vi "V3_IRCal.vi"() -> ()   [LabVIEW 2019]
uses:
  WSCbot_V3_Toolkit.lvlibp/WSCBOTV3_Toolkit/Sensor/LowLevel/IR_Chanel.ctl
  <vilib>/Platform/TimedLoop/XDataNode/timing_clust.ctl
  <vilib>/Platform/TimedLoop/XDataNode/nitl_modes.ctl
  <vilib>/Platform/TimedLoop/XDataNode/wakeup.ctl
  <vilib>/platform/TimedLoop/XDataNode/XDataNode.xnode
  WSCbot_V3_Toolkit.lvlibp
  <vilib>/Platform/TimedLoop/XDataNode/XDNodeRunTimeDep.lvlib
panel:
  out "x/y":dbl
  out "Waveform Chart 2":T1(graph)
  out "result":bool
  in  "P3":dbl
  in  "P2":dbl
  in  "P1":dbl
  out "Waveform Chart":T1(graph)
  in  "IR_Chanel":T2[](array[typedef])
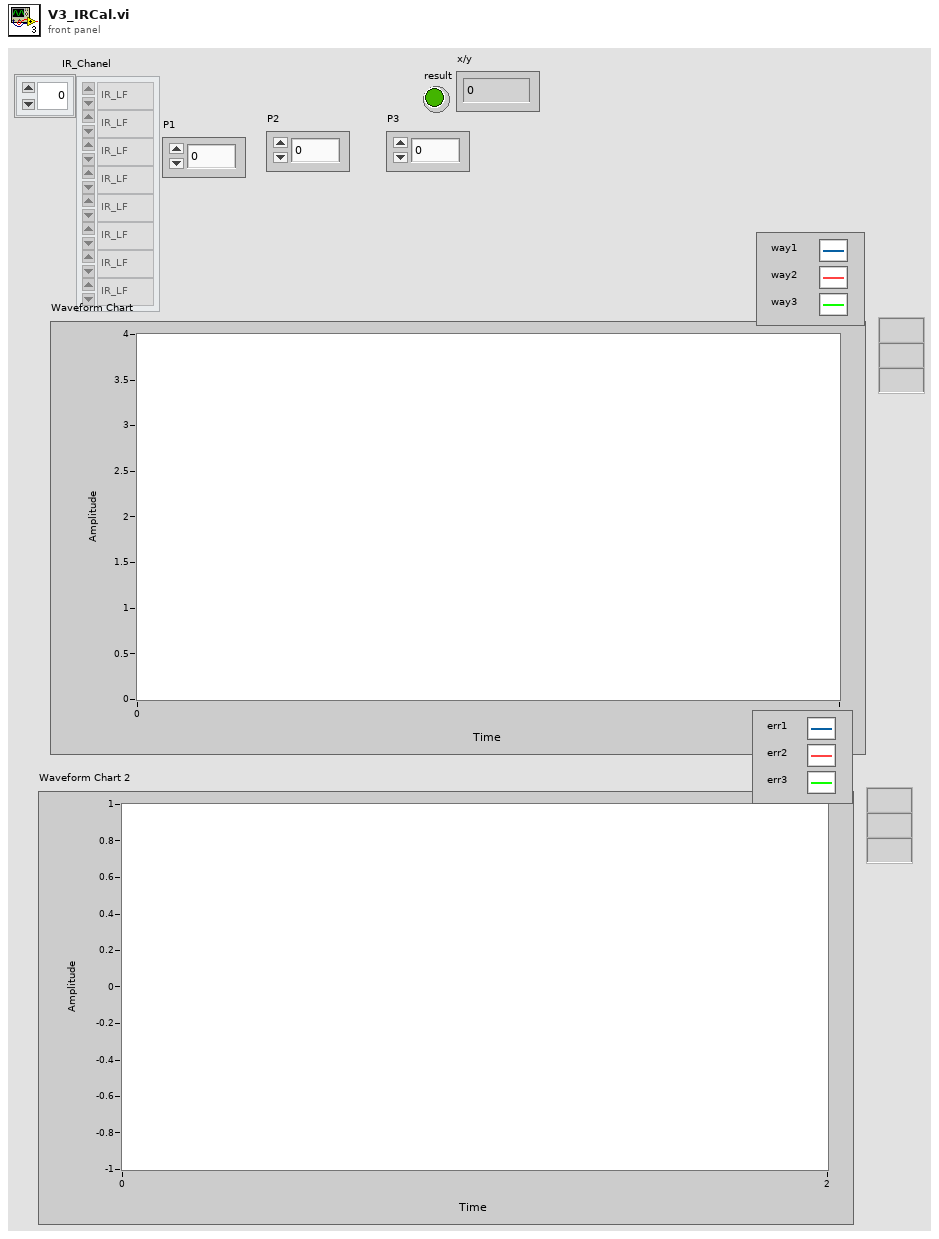
[diagram p1: front panel]
types:
  T1 = cluster{"Valtage[0]":dbl, "Valtage[1]":dbl, "Valtage[2]":dbl}
  T2 = typedef "WSCbot_V3_Toolkit.lvlibp/IR_Chanel.ctl" = enum16{"IR_LF", "IR_LB", "IR_BL", "IR_BR", "IR_RB", "IR_RF", "IR_FR", "IR_FL"}
  T3 = typedef "XDNodeRunTimeDep.lvlib/timing_clust.ctl" = cluster{"Expected End [f-1]":u64, "Actual End [f-1]":u64, "Finished Late? [f-1]":bool, "Expected End [i-1]":u64, "Actual End [i-1]":u64, "Finished Late? [i-1]":bool, "Expected Start [i]":u64, "Actual Start [i]":u64, "Expected Start [f]":u64, "Actual Start [f]":u64, "Source Name":string, "Structure Name":string, "Period":i64, "Deadline":i64, "Offset":i64, "Start":i64, "Priority":i32, "Timeout":i32, "Mode":T4, "Wakeup Reason":T5, "Error":errorcluster, "Source Type":string, "Secondary Source Type":string, "Global End Time":u64, "Global Start Time":u64, "Frame Duration":u64, "Iteration Duration":u64, "Assigned CPU":i32, "I/O Scan Engine Mode":u32}
  T4 = typedef "XDNodeRunTimeDep.lvlib/nitl_modes.ctl" = enum32{"No Change", "Process missed periods, maintain original phase", "Discard missed periods, maintain original phase", "Process missed periods, ignore original phase", "Discard missed periods, ignore original phase"}
  T5 = typedef "XDNodeRunTimeDep.lvlib/wakeup.ctl" = enum32{"Normal", "Aborted", "Asynchronous wakeup", "Timing source error", "Timed loop error", "Timeout"}
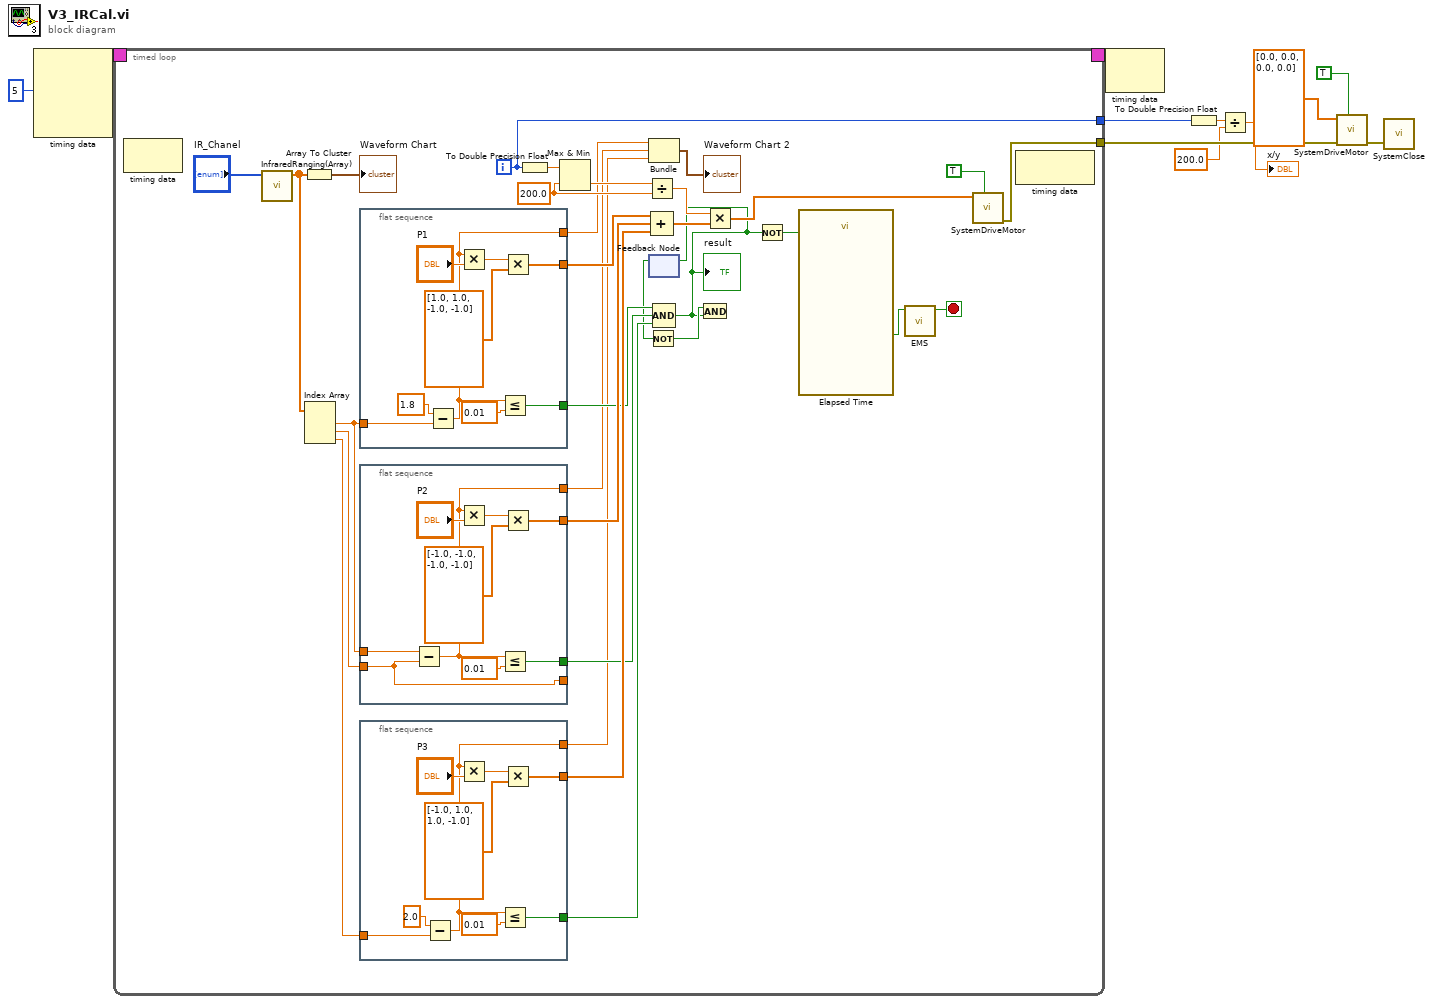
[diagram p0: block diagram]
diagram:
  n1 = node-c288(i64 5 ("Period")) -> (w11:T3)  [unwired: 3 in]
  n2 = timed-loop {
    timing: w11 -> [_]
    timing-out: [_] -> w10
    tunnel: [w33] -> w8
    tunnel: [w12] -> w4
    i -> [w12]
    stop <- w18 stop-if-true
    w28 = 200.0 ("y")
    n3 = node-c288() -> ()  [unwired: 1 in, 1 out]
    n4 = call "InfraredRanging(Array).vi"("IR_Chanel"="IR_Chanel") -> ("Valtage"=w40:dbl[])  [unwired: 9 in, 1 out]
    n5 = Array To Cluster(array=w40) -> (cluster=→"Waveform Chart":T1)
    n6 = Index Array(array=w40) -> (element #1=w37:dbl, element #2=w39:dbl, element #3=w38:dbl)  [unwired: 3 in]
    n7 = flat-sequence {
      tunnel: w37 -> [w68]
      tunnel: [w64] -> w36
      tunnel: [w62] -> w25
      tunnel: [w61] -> w15
      frame #0 {
        n8 = Subtract(x=1.8, y=w68) -> (x-y=w61:dbl)
        n9 = Multiply(x=w61, y="P1") -> (x*y=w66:dbl)
        n10 = Less Or Equal?(x=w61, y=0.01) -> (x <= y?=w62:bool)
        n11 = Multiply(x=w66, y=dbl[] [1.0, 1.0, -1.0, -1.0]) -> (x*y=w64:dbl[])
      }
    }
    n12 = flat-sequence {
      tunnel: [w59] -> _
      tunnel: w39 -> [w59]
      tunnel: w37 -> [w60]
      tunnel: [w55] -> w35
      tunnel: [w53] -> w24
      tunnel: [w52] -> w14
      frame #0 {
        n13 = Subtract(x=w60, y=w59) -> (x-y=w52:dbl)
        n14 = Multiply(x=w52, y="P2") -> (x*y=w56:dbl)
        n15 = Less Or Equal?(x=w52, y=0.01) -> (x <= y?=w53:bool)
        n16 = Multiply(x=w56, y=dbl[] [-1.0, -1.0, -1.0, -1.0]) -> (x*y=w55:dbl[])
      }
    }
    n17 = flat-sequence {
      tunnel: w38 -> [w51]
      tunnel: [w46] -> w26
      tunnel: [w44] -> w23
      tunnel: [w43] -> w13
      frame #0 {
        n18 = Subtract(x=2.0, y=w51) -> (x-y=w43:dbl)
        n19 = Multiply(x=w43, y="P3") -> (x*y=w48:dbl)
        n20 = Less Or Equal?(x=w43, y=0.01) -> (x <= y?=w44:bool)
        n21 = Multiply(x=w48, y=dbl[] [-1.0, 1.0, 1.0, -1.0]) -> (x*y=w46:dbl[])
      }
    }
    n22 = To Double Precision Float(number=w12) -> (double precision float=w30:dbl)
    n23 = Max & Min(x=w30, y=w28) -> (min(x,y)=w29:dbl)  [unwired: 1 out]
    n24 = Divide(x=w29, y=w28) -> (x/y=w27:dbl)
    n25 = Bundle(w15, w14, w13) -> (→"Waveform Chart 2":cluster{dbl, dbl, dbl})  [unwired: 1 in]
    n26 = feedback #1() -> (w22:bool)  [unwired: 1 in]
    n27 = Not(x=w22) -> (.not. x?=w21:bool)
    n28 = Compound Arithmetic op=ADD(w36, w35, w26) -> (w32:dbl[])
    n29 = Compound Arithmetic op=AND(w25, w24, w23) -> (w20:bool)
    "result" <- w20
    n30 = feedback-in #1(w20) -> ()
    n31 = And(x=w21, y=w20) -> ()  [unwired: 1 out]
    n32 = Multiply(x=w27, y=w32) -> (x*y=w31:dbl[])
    n33 = Not(x=w20) -> (.not. x?=w19:bool)
    n34 = call "Elapsed Time"("Reset"=w19) -> ("Time has Elapsed"=w17:bool)  [unwired: 11 in, 7 out]
    n35 = call "EMS.vi"("ProgramStop"=w17) -> ("EMS"=w18:bool)  [unwired: 9 in, 1 out]
    n36 = call "SystemDriveMotor.vi"("Enable?"=TRUE, "4xMotor(deg/s)"=w31) -> ("error out"=w33:errorcluster)  [unwired: 8 in, 1 out]
    n37 = node-c288() -> ()  [unwired: 1 in, 1 out]
  }
  n38 = node-c288(w10) -> ()  [unwired: 1 out]
  n39 = To Double Precision Float(number=w4) -> (double precision float=w3:dbl)
  n40 = Divide(x=w3, y=200.0) -> (x/y=→"x/y":dbl)
  n41 = call "SystemDriveMotor.vi"("Enable?"=TRUE, "error in"=w8, "4xMotor(deg/s)"=dbl[] [0.0, 0.0, 0.0, 0.0]) -> ("error out"=w5:errorcluster)  [unwired: 7 in, 1 out]
  n42 = call "SystemClose.vi"("error in"=w5) -> ()  [unwired: 2 in, 1 out]
